vi "Practica 4.vi"() -> ()   [LabVIEW 2020]
panel:
  out "Corriente":dynamicdata(graph)
  in  "?":bool
  out "Máximo":dbl
  out "Mínimo":dbl
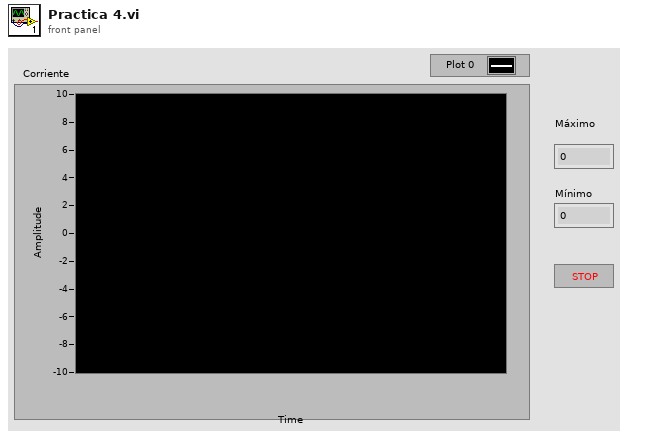
[diagram p1: front panel]
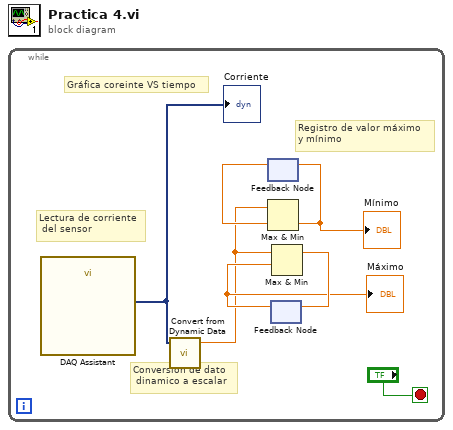
[diagram p0: block diagram]
diagram:
  n1 = while {
    stop <- "?" stop-if-true
    # "Conversión de dato\n dinamico a escalar"
    # "Registro de valor máximo\ny mínimo"
    # "Gráfica coreinte VS tiempo"
    # "Lectura de corriente\n del sensor"
    n2 = call "DAQ Assistant"() -> ("data"=w7:dynamicdata)  [unwired: 17 in, 2 out]
    "Corriente" <- w7
    n3 = call "Convert from Dynamic Data"("Dynamic Data Type"=w7) -> ("Scalar"=w1:dbl)  [unwired: 3 in]
    n4 = feedback #1() -> (w2:dbl)  [unwired: 1 in]
    n5 = Max & Min(x=w1, y=w2) -> (min(x,y)=w3:dbl)  [unwired: 1 out]
    "Mínimo" <- w3
    n6 = feedback-in #1(w3) -> ()
    n7 = feedback #2() -> (w4:dbl)  [unwired: 1 in]
    "Máximo" <- w4
    n8 = Max & Min(x=w1, y=w4) -> (max(x,y)=w5:dbl)  [unwired: 1 out]
    n9 = feedback-in #2(w5) -> ()
  }
